vi "DcMotorSim_Execute.vi"(5 "DCMotorSim_Model _Params":T2={"DCMOTOR_TYPES"=enum."NEO", "Num Motors"=1, "Gearing"=1.0, "MOI kgm2"=0.001} {"MOI kgm2" format="%#_13g"; "Gearing" format="%#_13g"}, 6 "dT_Seconds":dbl=0.02, 7 "DCMOTORSim_Simulation_Params":T1={"Pos Sim Std Dev Rotations"=2.0, "Vel Sim Std Dev RPM"=2.0} {"Vel Sim Std Dev RPM" format="%#_13g"; "Pos Sim Std Dev Rotations" format="%#_13g"}, 9 "Battery Voltage":dbl=12.0, 11 "Motor Dmd (CO)":dbl) -> (0 "Error":bool, 1 "Motor Current":dbl, 2 "Position_Rotations":dbl, 3 "Velocity_RPM":dbl, 4 "out DcMotorSim":T4 {"GearBox"."Jr_KgM2" format="%13.5p"; "GearBox"."L_H" format="%13.5p"; "GearBox"."Kt_NMPerAmp" format="%13.5p"; "GearBox"."KvINV_RadPerSecPerVolt" format="%13.5p"; "GearBox"."R_Ohms" format="%13.5p"; "GearBox"."FreeSpeed_RadPerSec" format="%13.5p"; "GearBox"."FreeCurrent_Amps" format="%13.5p"; "GearBox"."StallCurrent_Amps" format="%13.5p"; "GearBox"."StallTorque_NM" format="%13.5p"; "GearBox"."nominalVoltage_Volts" format="%13.5p"})   [LabVIEW 2019, in "Trajectory_Library.lvlib"]
uses:
  Trajectory_Library.lvlib
  TypeDef/DCMOTOR_SIM.ctl
  TypeDef/LINEAR_SYSTEM_SIM.ctl
  TypeDef/LINEAR_SYSTEM.ctl
  <vilib>/Analysis/Matrix/Datatypes/RealMatrix.ctl
  TypeDef/DCMOTOR.CTL
  TypeDef/LINEAR_SYSTEM_ID_DCMOTOR_MODEL.ctl
  Enum/DCMOTOR_TYPES_ENUM.ctl
  TypeDef/DCMOTOR_SIM_SIMULATION_PARAMS.ctl
  MatBuilder_Create.vi
  DCMotor_GetCIM.vi
  DCMotor_GetAndymark9015.vi
  DCMotor_GetAndymarkRs775_125.vi
  DCMotor_GetBag.vi
  DCMotor_GetBanebotsRs550.vi
  DCMotor_GetBanebotsRs775.vi
  DCMotor_GetFalcon500.vi
  DCMotor_GetMiniCIM.vi
  DCMotor_GetNEO.vi
  DCMotor_GetNEO550.vi
  DCMotor_GetRomiBuiltIn.vi
  DCMotor_GetVex775Pro.vi
  DCMotor_GetAndymarkAM2235A.vi
  DCMotor_GetAndymarkAM3493.vi
  LinearSystem_New.vi
  MatrixHelper_Zero.vi
  MatBuilder_Fill.vi
  Matrix_Ident.vi
  DCMotor_New.vi
  Units_RotationsPerMinuteToRadiansPerSecond.vi
  MatrixHelper_CoerceSize.vi
  <vilib>/Analysis/7linalg.llb/Create Special Matrix.vi
  <vilib>/Analysis/7linalg.llb/Create Special Real Matrix.vi
  <vilib>/Analysis/Matrix/NI_Matrix.lvlib
panel:
  # "<States, 1>"
  # "<Outputs, 1>"
  # "<Inputs, 1>"
  # "<Outputs, 1>"
  # "<States,States>"
  # "<States,Inputs>"
  # "<Outputs,States>"
  # "<Outputs,Inputs>"
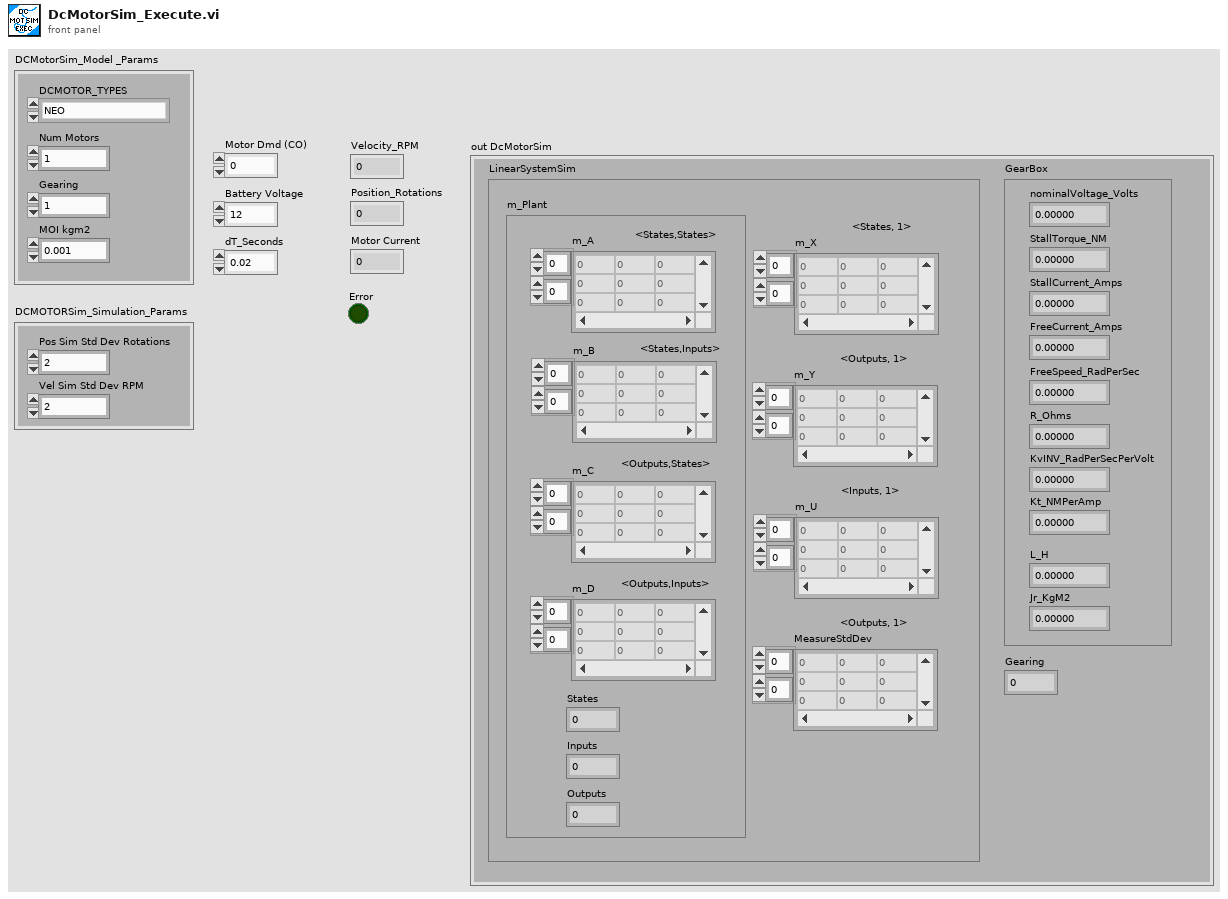
[diagram p1: front panel]
types:
  T1 = typedef "Trajectory_Library.lvlib/DCMOTOR_SIM_SIMULATION_PARAMS.ctl" = cluster{"Pos Sim Std Dev Rotations":dbl, "Vel Sim Std Dev RPM":dbl}
  T2 = typedef "Trajectory_Library.lvlib/LINEAR_SYSTEM_ID_DCMOTOR_MODEL.ctl" = cluster{"DCMOTOR_TYPES":T3, "Num Motors":i32, "Gearing":dbl, "MOI kgm2":dbl}
  T3 = typedef "Trajectory_Library.lvlib/DCMOTOR_TYPES_ENUM.ctl" = enum16{"CIM", "AndyMark 9015", "Andy Mark RS 775 125", "Bag", "BaneBots RS 550", "BaneBots RS 775", "Falcon 500", "Mini CIM", "NEO", "NEO 550", "Romi BuiltIn", "Vex 775 Pro", "Snow Blower AM 2235A", "Bosch Seat AM 3493"}
  T4 = typedef "Trajectory_Library.lvlib/DCMOTOR_SIM.ctl" = cluster{"LinearSystemSim":T5, "GearBox":T8, "Gearing":dbl}
  T5 = typedef "Trajectory_Library.lvlib/LINEAR_SYSTEM_SIM.ctl" = cluster{"m_Plant":T6, "m_X":T7, "m_Y":T7, "m_U":T7, "MeasureStdDev":T7}
  T6 = typedef "Trajectory_Library.lvlib/LINEAR_SYSTEM.ctl" = cluster{"m_A":T7, "m_B":T7, "m_C":T7, "m_D":T7, "States":i32, "Inputs":i32, "Outputs":i32}
  T7 = typedef "NI_Matrix.lvlib/RealMatrix.ctl" = dbl[][]
  T8 = typedef "Trajectory_Library.lvlib/DCMOTOR.CTL" = cluster{"nominalVoltage_Volts":dbl, "StallTorque_NM":dbl, "StallCurrent_Amps":dbl, "FreeCurrent_Amps":dbl, "FreeSpeed_RadPerSec":dbl, "R_Ohms":dbl, "KvINV_RadPerSecPerVolt":dbl, "Kt_NMPerAmp":dbl, "L_H":dbl, "Jr_KgM2":dbl}
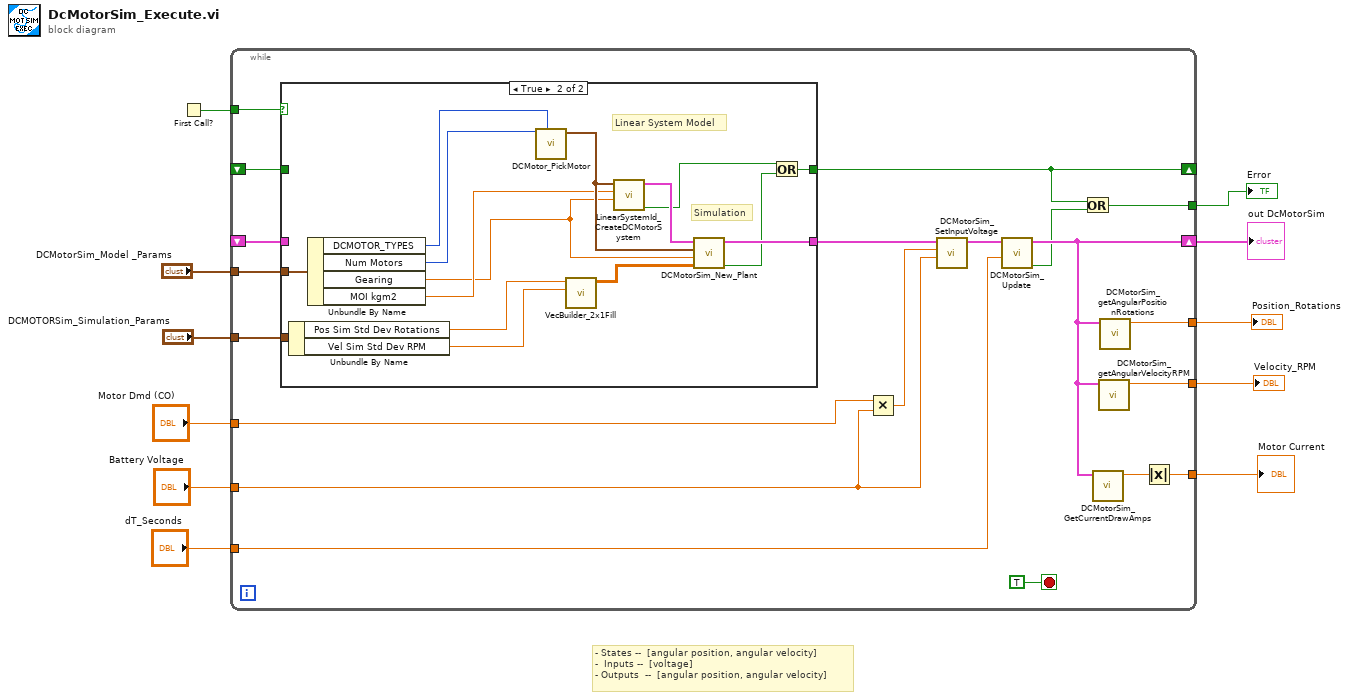
[diagram p0: block diagram]
diagram:
  # "- States --  [angular position, angular velocity]\n-  Inputs --  [voltage]\n- Outputs  --  [angular position, angular velocity]"
  n1 = First Call?() -> (First Call?: T/F=w7:bool)
  n2 = while {
    tunnel: "Motor Dmd (CO)" -> [w30]
    tunnel: "Battery Voltage" -> [w29]
    tunnel: "dT_Seconds" -> [w28]
    shift-right: [w19] -> w8
    shift-left: _ -> [w25]
    tunnel: w7 -> [w26]
    tunnel: "DCMotorSim_Model _Params" -> [w23]
    tunnel: [w20] -> w5
    tunnel: [w18] -> w4
    tunnel: [w17] -> w3
    shift-right: [w14] -> _
    shift-left: _ -> [w16]
    tunnel: [w13] -> w2
    tunnel: "DCMOTORSim_Simulation_Params" -> [w12]
    stop <- TRUE stop-if-true
    n3 = case shown="True" w26 {
      tunnel: w25 -> [w33 _]
      tunnel: [w33 w45] -> w24
      tunnel: w23 -> [_ w44]
      tunnel: [w32 w37] -> w14
      tunnel: w16 -> [w32 _]
      tunnel: w12 -> [_ w36]
      frame False {
      }
      frame True {
        # "Simulation"
        # "Linear System Model"
        n4 = Unbundle By Name(w36) -> ("Pos Sim Std Dev Rotations"=w35:dbl, "Vel Sim Std Dev RPM"=w34:dbl)
        n5 = Unbundle By Name(w44) -> ("DCMOTOR_TYPES"=w43:T3, "Num Motors"=w42:i32, "Gearing"=w40:dbl, "MOI kgm2"=w41:dbl)
        n6 = call "DCMotor_PickMotor.vi"("DCMOTOR_TYPES"=w43, "Num Motors"=w42) -> ("DCMOTOR"=w47:T8)  [unwired: 9 in]
        n7 = call "VecBuilder_2x1Fill.vi"("R1"=w34, "R0"=w35) -> ("output matrix"=w46:T7)  [unwired: 9 in]
        n8 = call "LinearSystemId_CreateDCMotorSystem.vi"("G"=w40, "jKgMetersSquared"=w41, "DCMOTOR"=w47) -> ("Error"=w38:bool, "Linearsystem"=w48:T6)  [unwired: 7 in]
        n9 = call "DCMotorSim_New_Plant.vi"("MeasurementStdDev"=w46, "Gearing"=w40, "GearBox"=w47, "Plant"=w48) -> ("Error"=w39:bool, "DCMotorSim"=w45:T4)  [unwired: 6 in]
        n10 = Or(x=w38, y=w39) -> (x .or. y?=w37:bool)
      }
    }
    n11 = Multiply(x=w30, y=w29) -> (x*y=w31:dbl)
    n12 = call "DCMotorSim_SetInputVoltage.vi"("Battery_Volts"=w29, "Volts"=w31, "DCMotorSim"=w24) -> ("out DCMotorSim"=w27:T4)  [unwired: 8 in]
    n13 = call "DCMotorSim_Update.vi"("dT_Seconds"=w28, "DCMotorSim"=w27) -> ("Error"=w15:bool, "out DCMotorSim"=w19:T4)  [unwired: 8 in]
    n14 = Or(x=w14, y=w15) -> (x .or. y?=w13:bool)
    n15 = call "DCMotorSim_GetCurrentDrawAmps.vi"("DCMotorSim"=w19) -> ("Current_Amps"=w21:dbl)  [unwired: 10 in]
    n16 = call "DCMotorSim_getAngularVelocityRPM.vi"("DCMotorSim"=w19) -> ("Velocity_RPM"=w18:dbl)  [unwired: 10 in]
    n17 = call "DCMotorSim_getAngularPositionRotations.vi"("DCMotorSim"=w19) -> ("Position_Rotations"=w17:dbl)  [unwired: 10 in]
    n18 = Absolute Value(x=w21) -> (abs(x)=w20:dbl)
  }
  "Motor Current" <- w5
  "out DcMotorSim" <- w8
  "Velocity_RPM" <- w4
  "Position_Rotations" <- w3
  "Error" <- w2
